vi "print pH.vi"(4 "gran":bool, 5 "Channel A":cluster{"time (s)":sgl[], "channel 1":dbl[]}(graph), 6 "Gran cluster":T1 {"r" format="%.4f"; "NC" format="%.3p"; "Ve" format="%.3f"; "Va" format="%.5f"; "F1" format="%.7f"}, 7 "units A":enum16{"OFF", "pH", "mV", "ion", "conductivity"}(ring)=enum."pH", 8 "Temperature":cluster{"time (s)":sgl[], "temperature":dbl[]}(graph), 9 "2nd channel":bool, 10 "units B":enum16{"OFF", "pH", "mV", "ion"}(ring)=enum."pH", 11 "Channel B":cluster{"time (s)":sgl[], "channel 2":dbl[]}(graph)) -> ()   [LabVIEW 2010]
panel:
  # "F1 vs. Titrant volume"
  # "mL"
  # "eq/L"
  # "titrant volume"
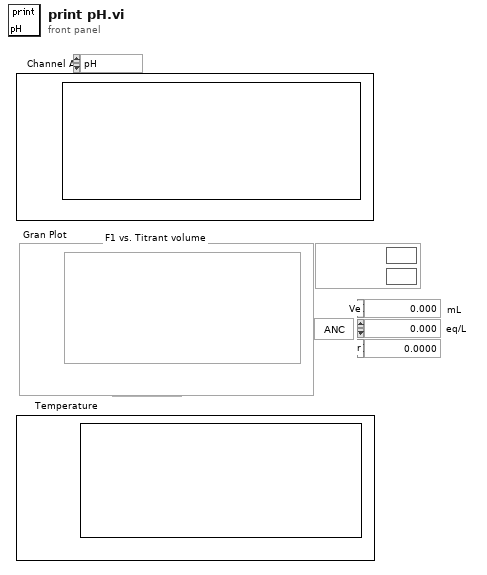
[diagram p1: front panel]
types:
  T1 = cluster{"F1":dbl[], "Va":dbl[], "Ve":dbl, "NC":dbl, "r":dbl, "Gran Plot":cluster{"Alkalinity":dbl[], "F1":dbl[]}[], "Measuring":bool}
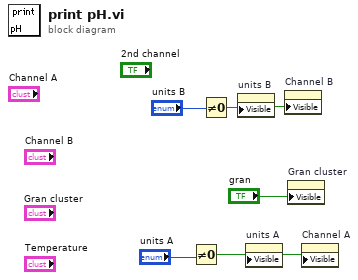
[diagram p0: block diagram]
diagram:
  n1 = Not Equal To 0?(x="units A") -> (x != 0?=w3:bool)
  n2 = Not Equal To 0?(x="units B") -> (x != 0?=w1:bool)
  n3 = property on="units B" class="Enum (strict)"("Visible"=w1) -> ()  [unwired: 2 in, 2 out]
  n4 = property on="units A" class="Enum (strict)"("Visible"=w3) -> ()  [unwired: 2 in, 2 out]
  n5 = property on="Channel B" class="XYGraph (strict)"("Visible"=w1) -> ()  [unwired: 2 in, 2 out]
  n6 = property on="Gran cluster" class="Clust (strict)"("Visible"="gran") -> ()  [unwired: 2 in, 2 out]
  n7 = property on="Channel A" class="XYGraph (strict)"("Visible"=w3) -> ()  [unwired: 2 in, 2 out]
